vi "Update.vi"(8 "error in (no error)":cluster{"状态":bool, "代码":i32, "源":string} caption="错误输入（无错误）", 11 "定时循环控制器输入":refnum<class "Timed Loop Actor.lvclass">) -> (0 "error out":cluster{"状态":bool, "代码":i32, "源":string} caption="错误输出", 3 "定时循环控制器输出":refnum<class "Timed Loop Actor.lvclass">)   [LabVIEW 2013, in "Timed Loop Actor.lvlib" / "Timed Loop Actor.lvclass"]
doc: "该VI对Update Core.vi进行包装，负责为Update Msg.lvclass:Do.vi提供库内范围接口。"
uses:
  Timed Loop Actor.lvclass
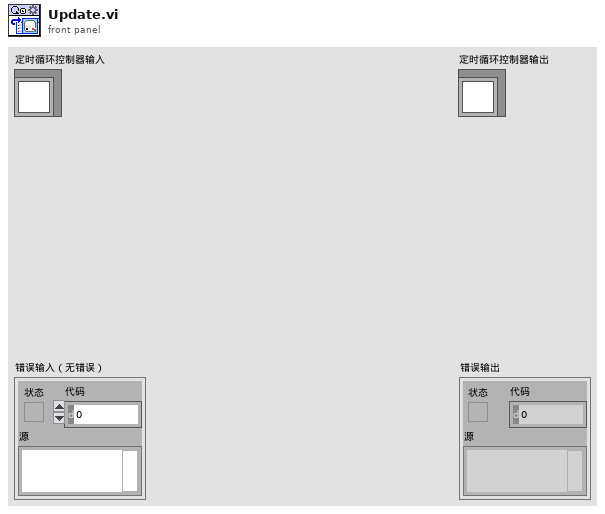
[diagram p1: front panel]
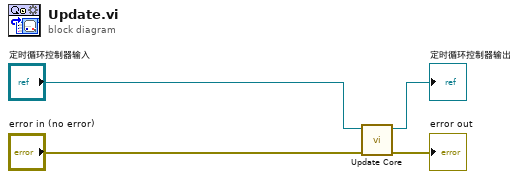
[diagram p0: block diagram]
diagram:
  n1 = call-dynamic "Update Core.vi"("error in (no error)"="error in (no error)", "水位控制器输入"="定时循环控制器输入") -> ("error out"=→"error out":cluster{"状态":bool, "代码":i32, "源":string}, "水位控制器输出"=→"定时循环控制器输出":refnum<class "Timed Loop Actor.lvclass">)  [unwired: 8 in]
